vi "Save Yield Counts.vi"(8 "error in (no error)":errorcluster, 10 "DatasFiles.DataWrite":variant, 11 "Master in":refnum<class "Master.lvclass">) -> (0 "error out":errorcluster, 3 "Master out":refnum<class "Master.lvclass">)   [LabVIEW 2014, in "Master.lvclass"]
uses:
  Master/Master.lvclass
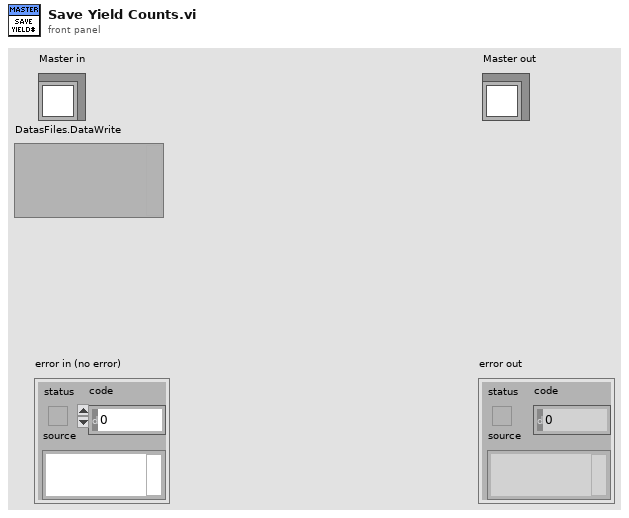
[diagram p1: front panel]
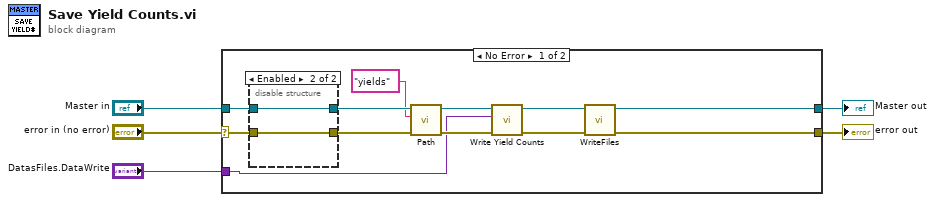
[diagram p0: block diagram]
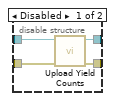
[diagram p2: hidden frame]
diagram:
  n1 = case shown="No Error" "error in (no error)" {
    selector: "error in (no error)" -> [w16 w25]
    tunnel: [w7 w25] -> w4
    tunnel: [w8 w24] -> w2
    tunnel: "Master in" -> [w17 w24]
    tunnel: "DatasFiles.DataWrite" -> [w6 _]
    frame No Error {
      n2 = disable-structure shown="Enabled" {
        disable-tunnel: w17 -> [w21 w23]
        disable-tunnel: w16 -> [w20 w22]
        disable-tunnel: [w19 w23] -> w15
        disable-tunnel: [w18 w22] -> w13
        frame Disabled {
          n3 = call-dynamic "Upload Yield Counts.vi"("error in (no error)"=w20, "Master in"=w21) -> ("error out"=w18:errorcluster, "Master out"=w19:refnum<class "Master.lvclass">)  [unwired: 8 in]
        }
        frame Enabled {
        }
      }
      n4 = call-dynamic "Path.vi"("error in (no error)"=w13, "pathname"="yields", "Master in"=w15) -> ("error out"=w11:errorcluster, "Master out"=w12:refnum<class "Master.lvclass">)  [unwired: 7 in]
      n5 = call-dynamic "Write Yield Counts.vi"("error in (no error)"=w11, "DatasFiles.DataWrite"=w6, "Master in"=w12) -> ("error out"=w10:errorcluster, "Master out"=w9:refnum<class "Master.lvclass">)  [unwired: 7 in]
      n6 = call-dynamic "WriteFiles.vi"("error in (no error)"=w10, "Master in"=w9) -> ("error out"=w7:errorcluster, "Master out"=w8:refnum<class "Master.lvclass">)  [unwired: 8 in]
    }
    frame Error {
    }
  }
  "error out" <- w4
  "Master out" <- w2
